vi "Multi_Trav_Move.vi"() -> ()   [LabVIEW 2022 SP3]
uses:
  Anemometry Sub Vis/Controls/User_Specific_mode.ctl
  Anemometry Sub Vis/Globals/Trav_pos_global.vi
  Anemometry Sub Vis/Gen Trav/Trav_mode.ctl
  Anemometry Sub Vis/Controls/Tunnel_Coordinates.ctl
  Anemometry Sub Vis/Globals/Constants_global.vi
  Anemometry Sub Vis/Gen Trav/Route mapping/Box_size.ctl
panel:
  in  "Live2":bool=TRUE
  in  "Live1":bool=TRUE
  in  "Mode":T1=enum."Read traverse position"
  in  "Offset on 2nd Traverse (Tun Cord)":sgl[](array[numeric])=[0.0, 0.0, 0.0] format="%.2f"
  out "Read Position 2":sgl[](array[numeric]) format="%#.2f"
  out "Read Position 1":sgl[](array[numeric]) format="%#.2f"
  out "XYZ 2":T2=[{"Max"=15.0, "Min"=-15.0}, {"Max"=250.0, "Min"=0.0}, {"Max"=15.0, "Min"=-15.0}] {"Min" format="%#.1f"; "Max" format="%#.1f"}
  out "Name2":string
  out "Probe Volume 2":T2=[{"Max"=15.0, "Min"=-15.0}, {"Max"=250.0, "Min"=0.0}, {"Max"=15.0, "Min"=-15.0}] {"Min" format="%#.1f"; "Max" format="%#.1f"}
  out "UW Offset Traverse Name":string
  out "UW Offset Position":sgl[](array[numeric]) format="%.2f"
  out "Probe Volume 1":T2=[{"Max"=15.0, "Min"=-15.0}, {"Max"=250.0, "Min"=0.0}, {"Max"=15.0, "Min"=-15.0}] {"Min" format="%#.1f"; "Max" format="%#.1f"}
  out "Name1":string
  out "XYZ 1":T2=[{"Max"=15.0, "Min"=-15.0}, {"Max"=250.0, "Min"=0.0}, {"Max"=15.0, "Min"=-15.0}] {"Min" format="%#.1f"; "Max" format="%#.1f"}
  in  "Work in Tunnel Coordinates?":T3
  out "Error String":string
  in  "Dem Position":sgl[](array[numeric])=[0.0, 0.0, 0.0] format="%#.2f"
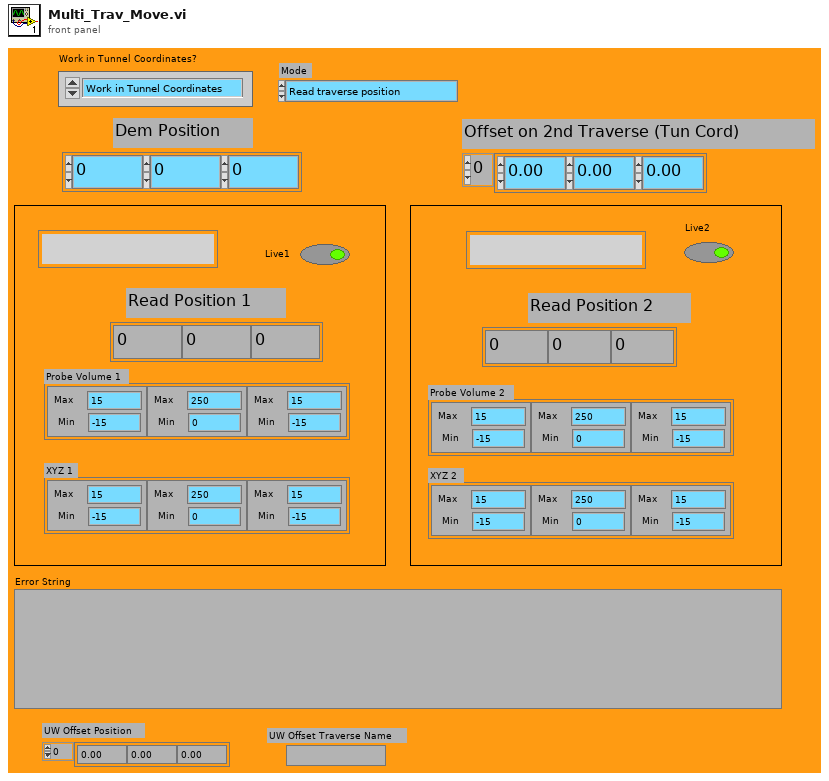
[diagram p1: front panel]
types:
  T1 = typedef "Trav_mode.ctl" = enum16{"Move traverse", "Read traverse position", "Teach Position"}
  T2 = typedef "Box_size.ctl" = cluster{"Max":sgl, "Min":sgl}[]
  T3 = typedef "Tunnel_Coordinates.ctl" = enum16{"Work in Tunnel Coordinates", "Work in Model Coordinates"}
  T4 = typedef "User_Specific_mode.ctl" = enum16{"Check VI only", "Run VI"}
  T5 = enum16{"To Traverse Coordinates", "To User Coordinates"}
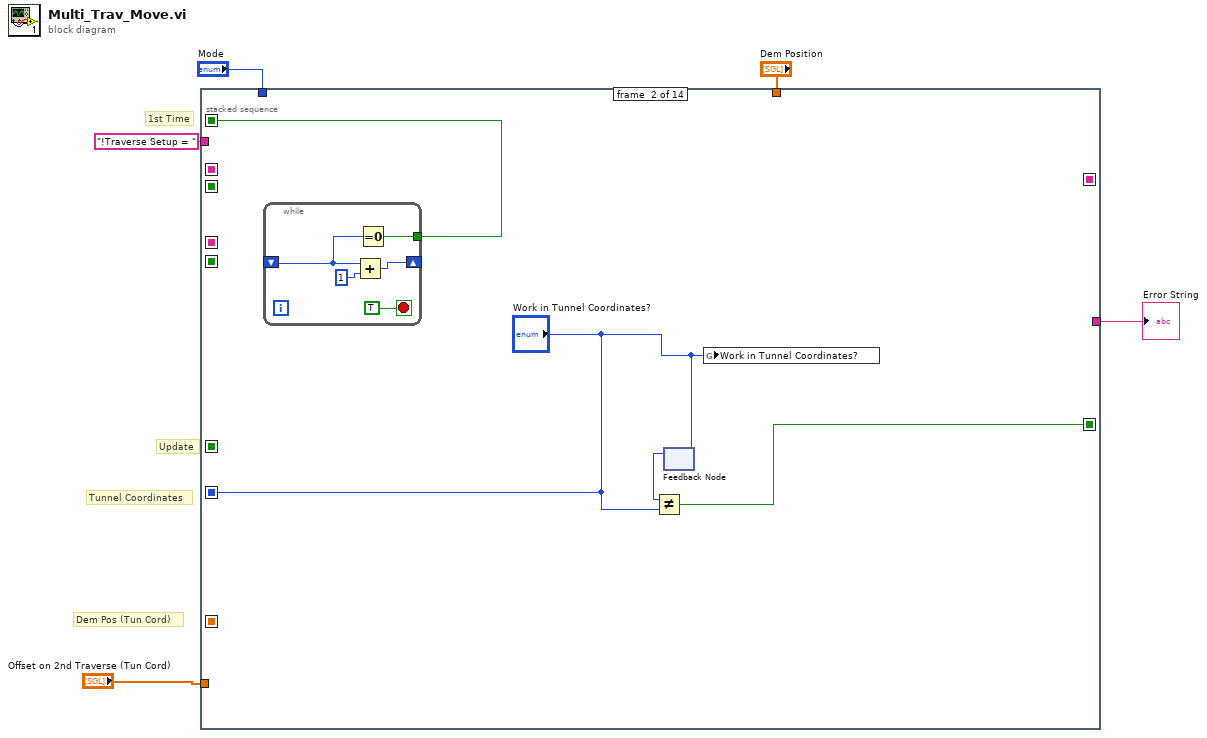
[diagram p0: block diagram]
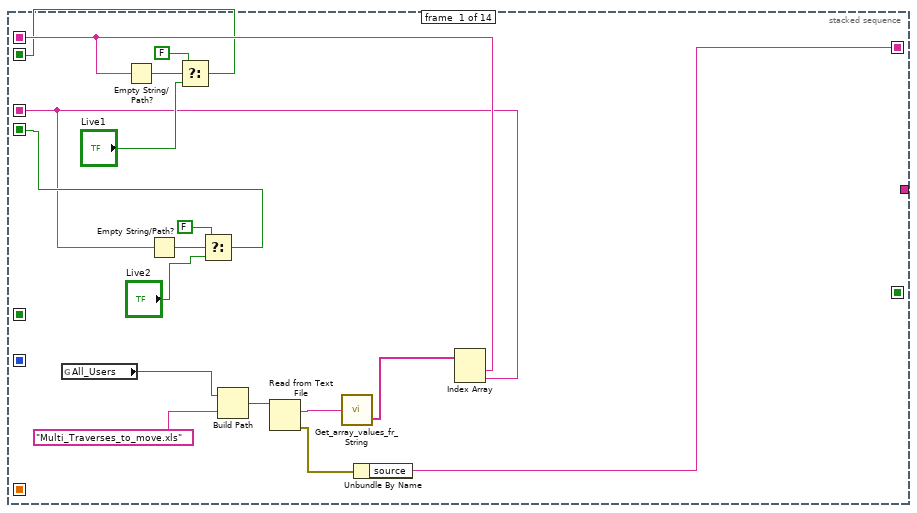
[diagram p2: hidden frame]
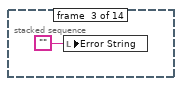
[diagram p3: hidden frame]
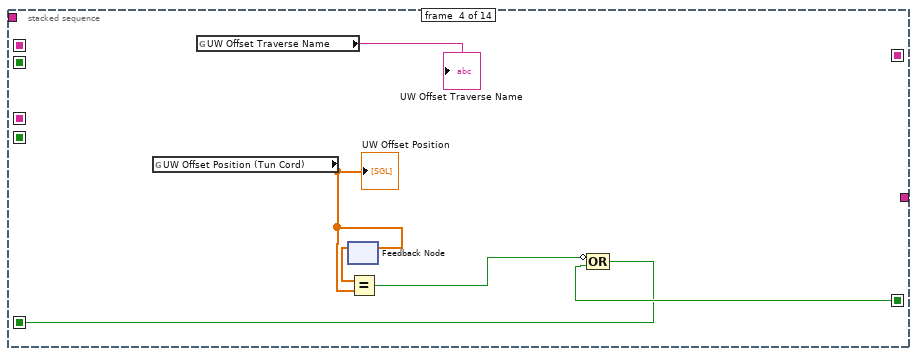
[diagram p4: hidden frame]
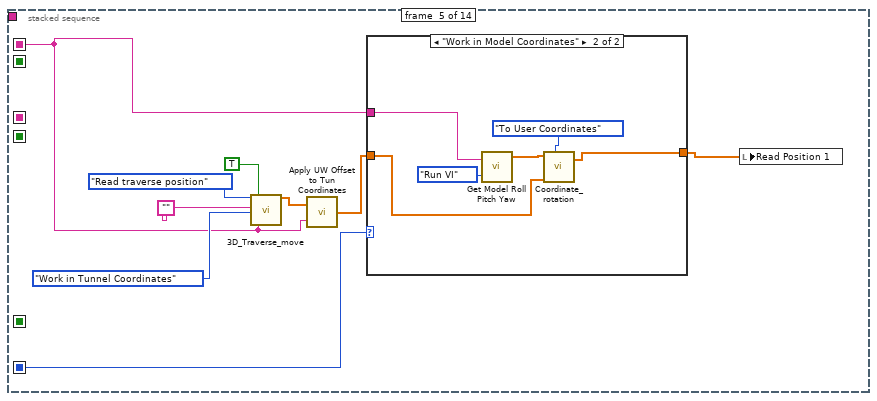
[diagram p5: hidden frame]
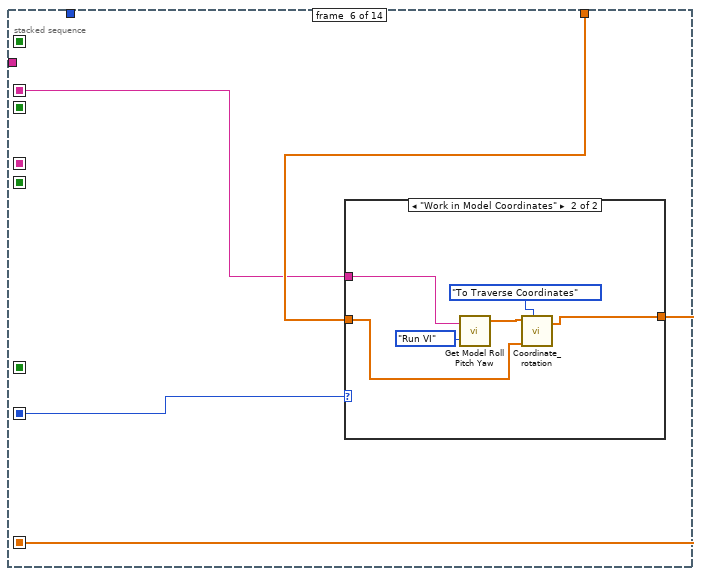
[diagram p7: hidden frame]
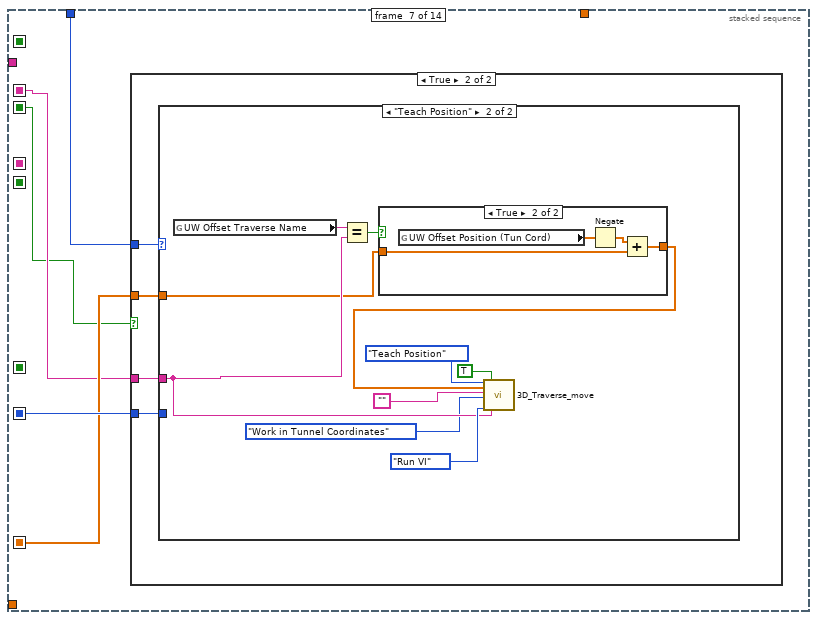
[diagram p9: hidden frame]
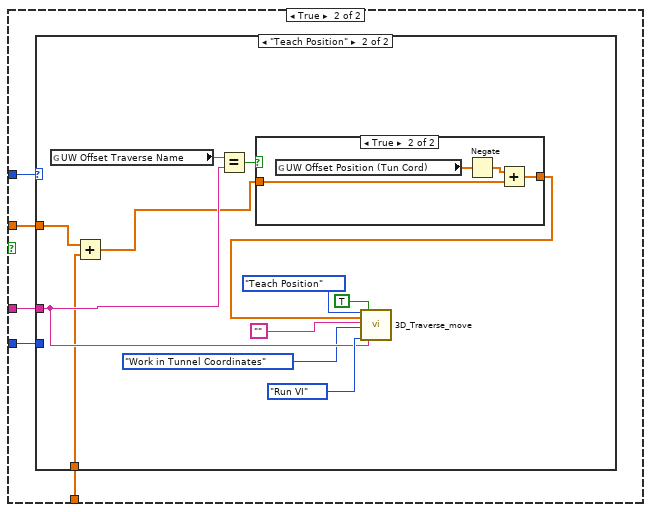
[diagram p14: hidden frame]
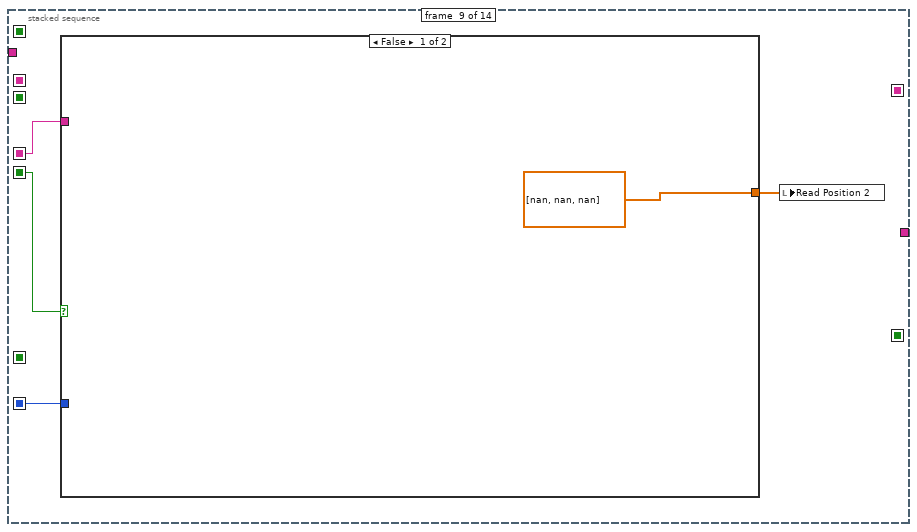
[diagram p17: hidden frame]
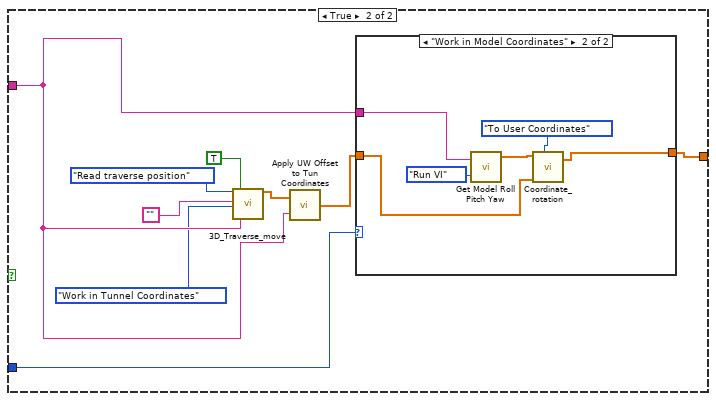
[diagram p18: hidden frame]
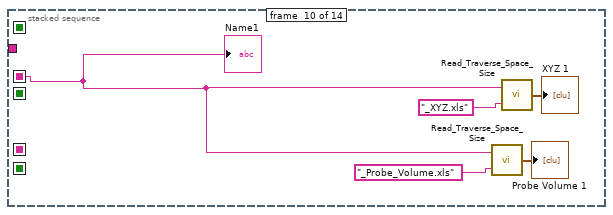
[diagram p20: hidden frame]
diagram:
  # "Dem Pos (Tun Cord)"
  # "Tunnel Coordinates"
  # "Update"
  # "1st Time"
  n1 = stacked-sequence {
    seq-local: [_ "Work in Tunnel Coordinates?" _ _ _ _ _ _ _ _ _ _ _ _] -> [_ _ _ _ w42 w58 w70 w95 w120 _ _ w197 _ w215]
    seq-local: [_ w26 _ _ _ _ _ _ _ _ _ _ _ _] -> [_ _ _ _ _ _ _ _ _ _ _ _ _ _]
    seq-local: [_ _ _ w33 _ _ _ _ _ _ _ _ _ _] -> [_ _ _ _ _ _ _ _ _ _ _ w190 _ _]
    seq-local: [_ w23 _ _ _ _ _ _ _ _ _ _ _ _] -> [_ _ _ w35 _ _ _ _ _ _ _ _ _ _]
    seq-local: [_ _ _ _ _ w56 _ _ _ _ _ _ _ _] -> [_ _ _ _ _ _ w68 w94 _ _ _ _ _ _]
    seq-local: [w17 _ _ _ _ _ _ _ _ _ _ _ _ _] -> [_ _ _ _ w39 w55 w67 _ _ w139 w150 w194 _ _]
    seq-local: [w8 _ _ _ _ _ _ _ _ _ _ _ _ _] -> [_ _ _ _ _ _ _ w90 w119 _ w149 _ w207 w213]
    seq-local: [w13 _ _ _ _ _ _ _ _ _ _ _ _ _] -> [_ _ _ _ _ _ w66 _ _ _ w148 _ _ _]
    seq-local: [w9 _ _ _ _ _ _ _ _ _ _ _ _ _] -> [_ _ _ _ _ _ _ w91 w118 _ w147 _ _ w212]
    seq-local: [w6 _ _ _ _ _ _ _ _ _ _ _ _ _] -> [_ _ _ _ _ _ _ _ _ _ w146 _ _ _]
    tunnel: "!Traverse Setup = " -> [_ _ _ _ _ _ _ _ _ _ _ _ _ _]
    tunnel: "Mode" -> [_ _ _ _ _ _ w69 w92 _ _ w154 _ _ _]
    tunnel: "Dem Position" -> [_ _ _ _ _ w57 _ _ _ _ w153 _ _ _]
    tunnel: "Offset on 2nd Traverse (Tun Cord)" -> [_ _ _ _ _ _ _ w93 _ _ w152 _ _ _]
    tunnel: [_ _ _ _ _ _ _ _ _ _ w144 _ _ _] -> w1
    frame #0 {
      n2 = global read "Constants_global.vi" "All_Users"() -> (w20:path)
      n3 = Build Path(base path=w20, name or relative path="Multi_Traverses_to_move.xls") -> (appended path=w21:path)
      n4 = Read from Text File(file (use dialog)=w21) -> (text=w19:string, error out=w7:errorcluster)  [unwired: 3 in, 2 out]
      n5 = call "Get_array_values_fr_String.vi"("String Value"=w19) -> ("String array"=w18:string[])  [unwired: 1 out]
      n6 = Unbundle By Name(w7) -> ("source"=w6:string)
      n7 = Index Array(array=w18) -> (element #1=w17:string, element #2=w8:string)  [unwired: 2 in]
      n8 = Empty String/Path?(string/path=w17) -> (empty?=w15:bool)
      n9 = Empty String/Path?(string/path=w8) -> (empty?=w11:bool)
      n10 = Select(t=FALSE, s=w15, f="Live1") -> (s? t:f=w13:bool)
      n11 = Select(t=FALSE, s=w11, f="Live2") -> (s? t:f=w9:bool)
    }
    frame #1 {
      n12 = while {
        shift-right: [w30] -> _
        shift-left: _ -> [w29]
        tunnel: [w28] -> w26
        stop <- TRUE stop-if-true
        n13 = Add(x=w29, y=1) -> (x+y=w30:i32)
        n14 = Equal To 0?(x=w29) -> (x = 0?=w28:bool)
      }
      n15 = feedback-in #1("Work in Tunnel Coordinates?") -> ()
      n16 = feedback #1() -> (w25:T3)  [unwired: 1 in]
      n17 = Not Equal?(x=w25, y="Work in Tunnel Coordinates?") -> (x != y?=w23:bool)
      n18 = global write "Trav_pos_global.vi" "Work in Tunnel Coordinates?"("Work in Tunnel Coordinates?") -> ()
    }
    frame #2 {
      n19 = local write "Error String"("") -> ()
    }
    frame #3 {
      n20 = global read "Trav_pos_global.vi" "UW Offset Position (Tun Cord)"() -> (w36:sgl[])
      "UW Offset Position" <- w36
      n21 = global read "Trav_pos_global.vi" "UW Offset Traverse Name"() -> (→"UW Offset Traverse Name":string)
      n22 = feedback-in #2(w36) -> ()
      n23 = feedback #2() -> (w37:sgl[])  [unwired: 1 in]
      n24 = Equal?(x=w37, y=w36) -> (x = y?=w34:bool)
      n25 = Compound Arithmetic op=OR(invert w34, w35) -> (w33:bool)
    }
    frame #4 {
      n26 = call "3D_Traverse_move.vi"("Mode"=Trav_mode."Read traverse position", "Extra command String"="", "Work in Tunnel Coordinates"=Tunnel_Coordinates."Work in Tunnel Coordinates", "Route Checking?"=TRUE, "Traverse name"=w39) -> ("Trav Position achieved"=w44:sgl[])  [unwired: 11 in, 3 out]
      n27 = call "Apply UW Offset to Tun Coordinates.vi"("Traverse Name"=w39, "Tunnel Coordinates"=w44) -> ("UW Offset Applied"=w43:sgl[])
      n28 = case shown="\"Work in Model Coordinates\"" w42 {
        tunnel: w43 -> [w48 w49]
        tunnel: w39 -> [_ w53]
        tunnel: [w48 w50] -> w47
        frame "Work in Tunnel Coordinates" {
        }
        frame "Work in Model Coordinates" {
          n29 = call "Get Model Roll Pitch Yaw.vi"("Traverse Name"=w53, "Mode"=User_Specific_mode."Run VI") -> ("Model:    Roll        Pitch         Yaw  (deg)"=w52:sgl[])  [unwired: 2 out]
          n30 = call "Coordinate_rotation.vi"("Roll-Pitch-Yaw"=w52, "Input Position"=w49, "Mode"=T5."To User Coordinates") -> ("Output Position"=w50:sgl[])  [unwired: 2 in, 1 out]
        }
      }
      n31 = local write "Read Position 1"(w47) -> ()
    }
    frame #5 {
      n32 = case shown="\"Work in Model Coordinates\"" w58 {
        tunnel: w57 -> [w59 w60]
        tunnel: w55 -> [_ w64]
        tunnel: [w59 w61] -> w56
        frame "Work in Tunnel Coordinates" {
        }
        frame "Work in Model Coordinates" {
          n33 = call "Get Model Roll Pitch Yaw.vi"("Traverse Name"=w64, "Mode"=User_Specific_mode."Run VI") -> ("Model:    Roll        Pitch         Yaw  (deg)"=w63:sgl[])  [unwired: 2 out]
          n34 = call "Coordinate_rotation.vi"("Roll-Pitch-Yaw"=w63, "Input Position"=w60, "Mode"=T5."To Traverse Coordinates") -> ("Output Position"=w61:sgl[])  [unwired: 2 in, 1 out]
        }
      }
    }
    frame #6 {
      n35 = case shown="True" w66 {
        tunnel: w67 -> [_ w74]
        tunnel: w70 -> [_ w73]
        tunnel: w69 -> [_ w72]
        tunnel: w68 -> [_ w71]
        frame False {
        }
        frame True {
          n36 = case shown="\"Teach Position\"" w72 {
            tunnel: w74 -> [_ w79]
            tunnel: w73 -> [_ _]
            tunnel: w71 -> [_ w76]
            frame "Move traverse", Default {
            }
            frame "Teach Position" {
              n37 = global read "Trav_pos_global.vi" "UW Offset Traverse Name"() -> (w84:string)
              n38 = Equal?(x=w84, y=w79) -> (x = y?=w83:bool)
              n39 = case shown="True" w83 {
                tunnel: [w85 w89] -> w81
                tunnel: w76 -> [w85 w86]
                frame False {
                }
                frame True {
                  n40 = global read "Trav_pos_global.vi" "UW Offset Position (Tun Cord)"() -> (w88:sgl[])
                  n41 = Negate(x=w88) -> (-x=w87:sgl[])
                  n42 = Add(x=w87, y=w86) -> (x+y=w89:sgl[])
                }
              }
              n43 = call "3D_Traverse_move.vi"("Mode"=Trav_mode."Teach Position", "Position"=w81, "Extra command String"="", "Work in Tunnel Coordinates"=Tunnel_Coordinates."Work in Tunnel Coordinates", "Simulate/Run"=User_Specific_mode."Run VI", "Route Checking?"=TRUE, "Traverse name"=w79) -> ()  [unwired: 9 in, 4 out]
            }
          }
        }
      }
    }
    frame #7 {
      n44 = case shown="False" w91 {
        tunnel: w95 -> [_ w100]
        tunnel: w94 -> [_ w99]
        tunnel: w93 -> [_ w98]
        tunnel: w90 -> [_ w97]
        tunnel: w92 -> [_ w96]
        frame False {
        }
        frame True {
          n45 = case shown="\"Teach Position\"" w96 {
            tunnel: w97 -> [_ w107]
            tunnel: w100 -> [_ _]
            tunnel: w99 -> [_ w104]
            tunnel: w98 -> [_ w103]
            frame "Move traverse", Default {
            }
            frame "Teach Position" {
              n46 = global read "Trav_pos_global.vi" "UW Offset Traverse Name"() -> (w112:string)
              n47 = Add(x=w104, y=w103) -> (x+y=w102:sgl[])
              n48 = Equal?(x=w112, y=w107) -> (x = y?=w111:bool)
              n49 = case shown="True" w111 {
                tunnel: [w113 w117] -> w109
                tunnel: w102 -> [w113 w114]
                frame False {
                }
                frame True {
                  n50 = global read "Trav_pos_global.vi" "UW Offset Position (Tun Cord)"() -> (w116:sgl[])
                  n51 = Negate(x=w116) -> (-x=w115:sgl[])
                  n52 = Add(x=w115, y=w114) -> (x+y=w117:sgl[])
                }
              }
              n53 = call "3D_Traverse_move.vi"("Mode"=Trav_mode."Teach Position", "Position"=w109, "Extra command String"="", "Work in Tunnel Coordinates"=Tunnel_Coordinates."Work in Tunnel Coordinates", "Simulate/Run"=User_Specific_mode."Run VI", "Route Checking?"=TRUE, "Traverse name"=w107) -> ()  [unwired: 9 in, 4 out]
            }
          }
        }
      }
    }
    frame #8 {
      n54 = case shown="False" w118 {
        tunnel: [sgl[] [nan, nan, nan] ("Output Position") w131] -> w121
        tunnel: w119 -> [_ w127]
        tunnel: w120 -> [_ w125]
        frame False {
        }
        frame True {
          n55 = call "3D_Traverse_move.vi"("Mode"=Trav_mode."Read traverse position", "Extra command String"="", "Work in Tunnel Coordinates"=Tunnel_Coordinates."Work in Tunnel Coordinates", "Route Checking?"=TRUE, "Traverse name"=w127) -> ("Trav Position achieved"=w128:sgl[])  [unwired: 11 in, 3 out]
          n56 = call "Apply UW Offset to Tun Coordinates.vi"("Traverse Name"=w127, "Tunnel Coordinates"=w128) -> ("UW Offset Applied"=w126:sgl[])
          n57 = case shown="\"Work in Model Coordinates\"" w125 {
            tunnel: w126 -> [w132 w133]
            tunnel: w127 -> [_ w137]
            tunnel: [w132 w134] -> w131
            frame "Work in Tunnel Coordinates" {
            }
            frame "Work in Model Coordinates" {
              n58 = call "Get Model Roll Pitch Yaw.vi"("Traverse Name"=w137, "Mode"=User_Specific_mode."Run VI") -> ("Model:    Roll        Pitch         Yaw  (deg)"=w136:sgl[])  [unwired: 2 out]
              n59 = call "Coordinate_rotation.vi"("Roll-Pitch-Yaw"=w136, "Input Position"=w133, "Mode"=T5."To User Coordinates") -> ("Output Position"=w134:sgl[])  [unwired: 2 in, 1 out]
            }
          }
        }
      }
      n60 = local write "Read Position 2"(w121) -> ()
    }
    frame #9 {
      n61 = call "Read_Traverse_Space_Size.vi"("Space_Name"="_Probe_Volume.xls" ("string"), "Traverse Name"=w139) -> ("Limits out"=→"Probe Volume 1":T2)
      n62 = call "Read_Traverse_Space_Size.vi"("Space_Name"="_XYZ.xls" ("string"), "Traverse Name"=w139) -> ("Limits out"=→"XYZ 1":T2)
      "Name1" <- w139
    }
    frame #10 {
      n63 = Equal?(x=Trav_mode."Move traverse" ("Mode 1"), y=w154) -> (x = y?=w151:bool)
      n64 = case shown="True" w151 {
        tunnel: w150 -> [_ w172]
        tunnel: w149 -> [_ w169]
        tunnel: ["" w161] -> w145
        tunnel: w153 -> [_ w160]
        tunnel: w152 -> [_ w159]
        tunnel: w147 -> [_ w158]
        tunnel: w148 -> [_ w157]
        frame False {
        }
        frame True {
          n65 = case shown="True" w157 {
            tunnel: w172 -> [_ w187]
            tunnel: ["" w186] -> w170
            frame False {
            }
            frame True {
              n66 = Concatenate Strings(w187, "; " ("string")) -> (w186:string)
            }
          }
          n67 = case shown="True" w158 {
            tunnel: w169 -> [_ w183]
            tunnel: ["" w182] -> w168
            frame False {
            }
            frame True {
              n68 = Concatenate Strings(w183, "; " ("string")) -> (w182:string)
            }
          }
          n69 = And(x=w157, y=w158) -> (x .and. y?=w164:bool)
          n70 = Number To Fractional String(number=w159, precision (6)=i16 1) -> (F-format string=w166:string[])  [unwired: 2 in]
          n71 = Concatenate Strings("!Traverse Setup = ", w170, w168) -> (w165:string)
          n72 = case shown="True" w164 {
            tunnel: w166 -> [_ w176]
            tunnel: w165 -> [w173 w175]
            tunnel: [w173 w174] -> w163
            frame False {
            }
            frame True {
              n73 = for {
                shift-right: [w177] -> w174
                shift-left: w175 -> [w180]
                tunnel: w176 -> [w179] mode=indexing
                n74 = Concatenate Strings(w180, w179, ";") -> (w177:string)
              }
            }
          }
          n75 = call "2_Trav_move.vi"("Extra Command String"=w163, "New Position"=w160, "Simulate/Run"=User_Specific_mode."Run VI") -> ("Error String"=w161:string)  [unwired: 10 in, 2 out]
        }
      }
      n76 = Concatenate Strings(w146, w145) -> (w144:string)
    }
    frame #11 {
      n77 = call "Read-Write_Check_Pos.vi"("Mode"=enum16{"Read", "Write"}."Read", "Traverse Name"=w194) -> ("Position Output with UW Offset"=w196:sgl[])  [unwired: 3 in, 2 out]
      n78 = case shown="\"Work in Model Coordinates\"" w197 {
        tunnel: w196 -> [w200 w201]
        tunnel: w194 -> [_ w205]
        tunnel: [w200 w202] -> w195
        frame "Work in Tunnel Coordinates" {
        }
        frame "Work in Model Coordinates" {
          n79 = call "Get Model Roll Pitch Yaw.vi"("Traverse Name"=w205, "Mode"=User_Specific_mode."Run VI") -> ("Model:    Roll        Pitch         Yaw  (deg)"=w204:sgl[])  [unwired: 2 out]
          n80 = call "Coordinate_rotation.vi"("Roll-Pitch-Yaw"=w204, "Input Position"=w201, "Mode"=T5."To User Coordinates") -> ("Output Position"=w202:sgl[])  [unwired: 2 in, 1 out]
        }
      }
      "Read Position 1" <- w195
      n81 = local read "Dem Position"() -> (w193:sgl[])
      n82 = Array Size(array=w193) -> (size(s)=w192:i32)
      n83 = Equal To 0?(x=w192) -> (x = 0?=w191:bool)
      n84 = Or(x=w190, y=w191) -> (x .or. y?=w189:bool)
      n85 = case shown="True" w189 {
        tunnel: w195 -> [_ w199]
        frame False {
        }
        frame True {
          n86 = local write "Dem Position"(w199) -> ()
        }
      }
    }
    frame #12 {
      n87 = call "Read_Traverse_Space_Size.vi"("Space_Name"="_Probe_Volume.xls" ("string"), "Traverse Name"=w207) -> ("Limits out"=→"Probe Volume 2":T2)
      n88 = call "Read_Traverse_Space_Size.vi"("Space_Name"="_XYZ.xls" ("string"), "Traverse Name"=w207) -> ("Limits out"=→"XYZ 2":T2)
      "Name2" <- w207
    }
    frame #13 {
      n89 = case shown="False" w212 {
        tunnel: w215 -> [_ w220]
        tunnel: w213 -> [_ w218]
        tunnel: [sgl[] [nan, nan, nan] ("Output Position") w217] -> w214
        frame False {
        }
        frame True {
          n90 = call "Read-Write_Check_Pos.vi"("Mode"=enum16{"Read", "Write"}."Read", "Traverse Name"=w218) -> ("Position Output with UW Offset"=w219:sgl[])  [unwired: 3 in, 2 out]
          n91 = case shown="\"Work in Model Coordinates\"" w220 {
            tunnel: w219 -> [w222 w223]
            tunnel: w218 -> [_ w227]
            tunnel: [w222 w224] -> w217
            frame "Work in Tunnel Coordinates" {
            }
            frame "Work in Model Coordinates" {
              n92 = call "Get Model Roll Pitch Yaw.vi"("Traverse Name"=w227, "Mode"=User_Specific_mode."Run VI") -> ("Model:    Roll        Pitch         Yaw  (deg)"=w226:sgl[])  [unwired: 2 out]
              n93 = call "Coordinate_rotation.vi"("Roll-Pitch-Yaw"=w226, "Input Position"=w223, "Mode"=T5."To User Coordinates") -> ("Output Position"=w224:sgl[])  [unwired: 2 in, 1 out]
            }
          }
        }
      }
      "Read Position 2" <- w214
    }
  }
  "Error String" <- w1
